vi "Delete RT FIFO.vi"   [LabVIEW 2017, in "Data Sharing Framework Core.lvlib" / "Data Sharing Framework Engine.lvlib" / "Engine Interface.lvclass"]
uses:
  Engine Interface.lvclass
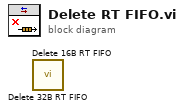
[diagram p0: block diagram]
diagram:
  n1 = call "Delete 32B RT FIFO.vi"() -> ()  [unwired: 11 in, 1 out]
  n2 = call "Delete 16B RT FIFO.vi"() -> ()  [unwired: 11 in, 1 out]
